vi "Create Notifier for Simulated Data.vi"(8 "error in (no error)":errorcluster) -> (0 "error out":errorcluster, 3 "Notifier out":refnum<notifier>)   [LabVIEW 2020]
doc: "Creates the notifier for the display. Since a notifier is a potentially lossy communication mechanism, it is acceptable to use for data display, but not for logging."
uses:
  controls/Simulated Data.ctl
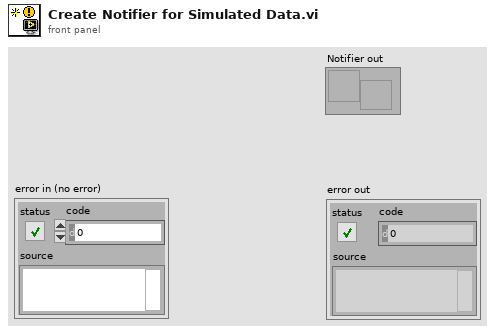
[diagram p1: front panel]
types:
  T1 = typedef "Simulated Data.ctl" = cluster{"temperature":dbl, "High Limit":dbl, "Low Limit":dbl}
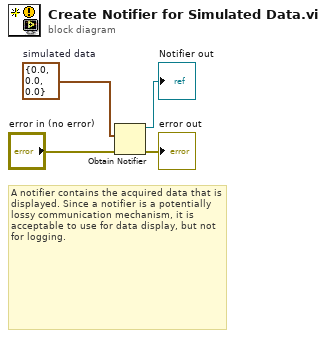
[diagram p0: block diagram]
diagram:
  w4 = T1 {"temperature"=0.0, "High Limit"=0.0, "Low Limit"=0.0}  # simulated data
  # "A notifier contains the acquired data that is displayed. Since a notifier is a potentially lossy communication mechanism, it is acceptable to use for data display, but not for logging."
  n1 = Obtain Notifier(notification data type=w4, error in (no error)="error in (no error)") -> (notifier out=→"Notifier out":refnum<notifier>, error out=→"error out":errorcluster)  [unwired: 2 in, 1 out]
